vi "ArduinoLT_Config.vi"(5 "error in":errorcluster, 8 "VISA resource":refnum<visa-resource-name>) -> (0 "error out":errorcluster, 1 "Thermometer [C]":dbl(slide) scale=0.0..50.0, 2 "Arduino Configuration OUT":T2={"Lights: Digital I/O Pins"={"Coaxial"=0, "Spotlights"=0}, "Thermistor Settings"={"Analogue Readout Pin"=1, "Vcc Reference Pin"=0, "Paired Resistance (10K Ohms)"=10000.0, "Units (C)"=enum."Celsius"}} {"Thermistor Settings"."Paired Resistance (10K Ohms)" format="%#_13g"}, 3 "Arduino Resource":T3={"VISA resource"="COM11", "Board Type"=enum."Uno", "Connection Type"=enum."USB / Serial", "Bytes Per Packet (15)"=15})   [LabVIEW 2016]
uses:
  <vilib>/LabVIEW Interface for Arduino/Type Defs/Arduino Resource.ctl
  <vilib>/LabVIEW Interface for Arduino/Type Defs/Board Type.ctl
  Controls/ArduinoLT-ConfigurationControl.ctl
  <vilib>/LabVIEW Interface for Arduino/Type Defs/Pin Mode.ctl
  <vilib>/LabVIEW Interface for Arduino/LabVIEW Interface for Arduino.lvlib
panel:
  in  "Tab Control":T1(tab)
  in  "Arduino Configuration":T2={"Lights: Digital I/O Pins"={"Coaxial"=6, "Spotlights"=5}, "Thermistor Settings"={"Analogue Readout Pin"=1, "Vcc Reference Pin"=0, "Paired Resistance (10K Ohms)"=10000.0, "Units (C)"=enum."Celsius"}} {"Thermistor Settings"."Paired Resistance (10K Ohms)" format="%#_13g"}
  out "VCC [V]":dbl=5.0 format="%#_13g"
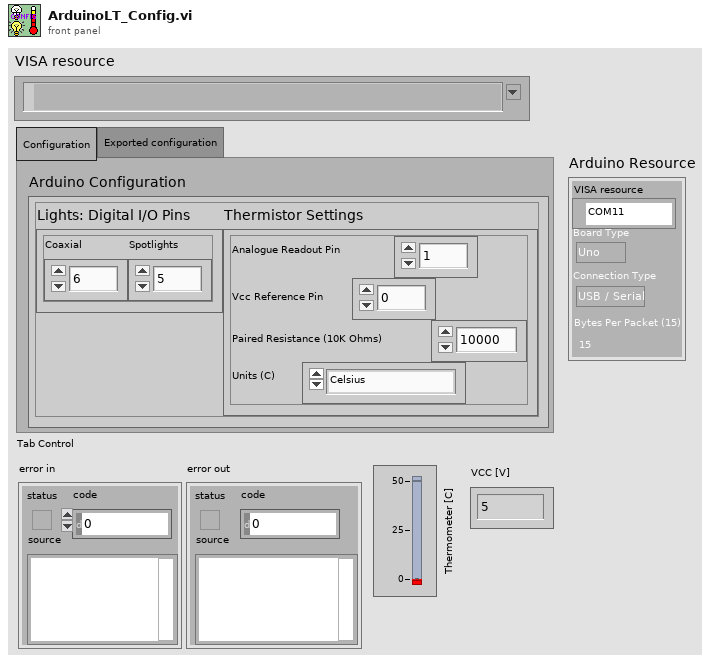
[diagram p1: front panel]
types:
  T1 = enum32{"Configuration", "Exported configuration"}
  T2 = typedef "ArduinoLT-ConfigurationControl.ctl" = cluster{"Lights: Digital I/O Pins":cluster{"Coaxial":u8, "Spotlights":u8}, "Thermistor Settings":cluster{"Analogue Readout Pin":u8, "Vcc Reference Pin":u8, "Paired Resistance (10K Ohms)":dbl, "Units (C)":enum16{"Celsius", "Fahrenheit", "Kelvin"}}}
  T3 = typedef "LabVIEW Interface for Arduino.lvlib/Arduino Resource.ctl" = cluster{"VISA resource":refnum<visa-resource-name>, "Board Type":T4, "Connection Type":enum8{"USB / Serial"}, "Bytes Per Packet (15)":u8}
  T4 = typedef "LabVIEW Interface for Arduino.lvlib/Board Type.ctl" = enum16{"Uno", "Dimuelanove w/Atmega 328", "Mega 2560"}
  T5 = typedef "LabVIEW Interface for Arduino.lvlib/Pin Mode.ctl" = enum8{"Input", "Output"}
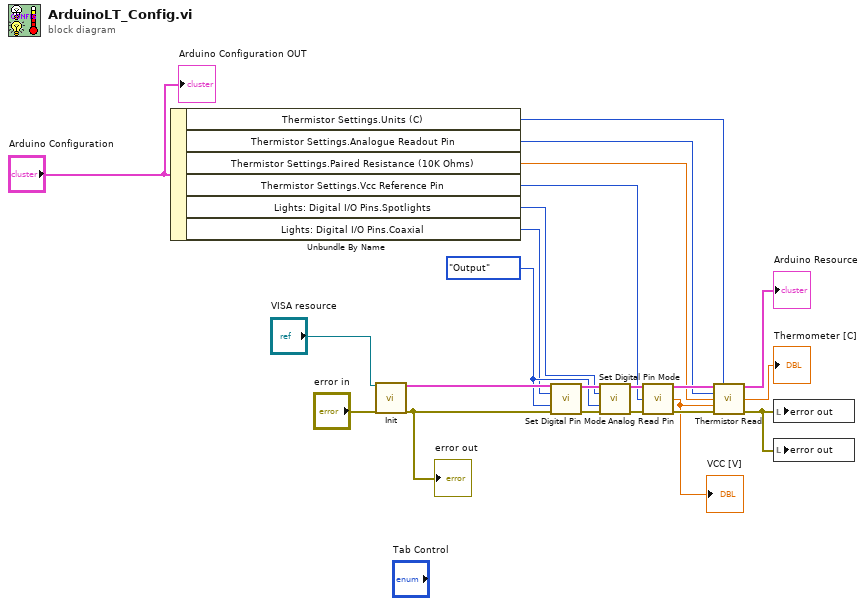
[diagram p0: block diagram]
diagram:
  w16 = Pin_Mode."Output" ("Pin Mode (Input)")
  n1 = Unbundle By Name("Arduino Configuration") -> ("Thermistor Settings.Units (C)"=w2:enum16{"Celsius", "Fahrenheit", "Kelvin"}, "Thermistor Settings.Analogue Readout Pin"=w3:u8, "Thermistor Settings.Paired Resistance (10K Ohms)"=w4:dbl, "Thermistor Settings.Vcc Reference Pin"=w5:u8, "Lights: Digital I/O Pins.Spotlights"=w6:u8, "Lights: Digital I/O Pins.Coaxial"=w7:u8)
  n2 = call <vilib>:"Init.vi"("VISA resource"="VISA resource", "error in"="error in") -> ("Arduino Resource"=w20:T3, "error out"=w14:errorcluster)  [unwired: 16 in]
  "error out" <- w14
  n3 = call <vilib>:"Set Digital Pin Mode.vi"("Arduino Resource"=w20, "Digital I/O Pin"=w7, "Pin Mode (Input)"=w16, "error in"=w14) -> ("Arduino Resource"=w18:T3, "error out"=w17:errorcluster)  [unwired: 10 in]
  n4 = call <vilib>:"Set Digital Pin Mode.vi"("Arduino Resource"=w18, "Digital I/O Pin"=w6, "Pin Mode (Input)"=w16, "error in"=w17) -> ("Arduino Resource"=w10:T3, "error out"=w9:errorcluster)  [unwired: 10 in]
  n5 = call <vilib>:"Analog Read Pin.vi"("Arduino Resource"=w10, "Analog Input Pin (0)"=w5, "error in"=w9) -> ("Arduino Resource"=w13:T3, "Voltage"=w11:dbl, "error out"=w12:errorcluster)  [unwired: 10 in]
  "VCC [V]" <- w11
  n6 = call <vilib>:"Thermistor Read.vi"("Arduino Resource"=w13, "Units (C)"=w2, "Thermistor AI Pin (0)"=w3, "Paired Resistance (10K Ohms)"=w4, "Vcc (5 v)"=w11, "error in"=w12) -> ("Arduino Resource"=→"Arduino Resource":T3, "Temperature"=→"Thermometer [C]":dbl, "error out"=w19:errorcluster)  [unwired: 7 in]
  n7 = local write "error out"(w19) -> ()
  n8 = local write "error out"(w19) -> ()
  "Arduino Configuration OUT" <- "Arduino Configuration"
